vi "Calculate Indices.vi"(8 "Cursor.Cursor Y":dbl, 9 "Cursor.Cursor X":dbl, 10 "Vslow":dbl[](array[numeric]), 11 "Vfast":dbl[][](array[numeric])) -> (0 "Column":i32, 1 "Row":i32, 2 "Column Array":i32[](array[numeric]), 3 "Row Array":i32[](array[numeric]))   [LabVIEW 2016, in "Retrieve and Visualize.lvclass"]
uses:
  Retrieve and Visualize.lvclass
  <vilib>/gmath/NI_Gmath.lvlib
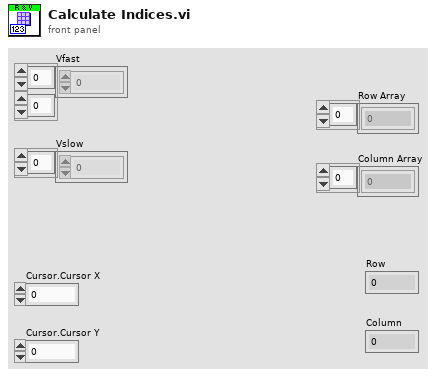
[diagram p1: front panel]
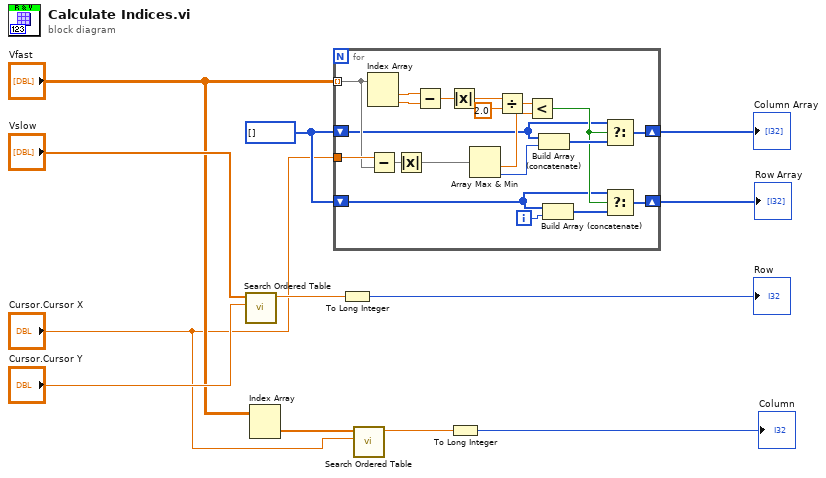
[diagram p0: block diagram]
diagram:
  w10 = i32[] []
  n1 = call <vilib>:"Search Ordered Table.vi"("x value"="Cursor.Cursor Y", "ordered x array"="Vslow") -> ("fractional index"=w6:dbl)  [unwired: 9 in]
  n2 = Index Array(array="Vfast") -> (element=w4:dbl[])  [unwired: 2 in]
  n3 = for {
    tunnel: "Vfast" -> [w15] mode=indexing
    tunnel: "Cursor.Cursor X" -> [w29]
    shift-right: [w21] -> w9
    shift-left: w10 -> [w14]
    shift-right: [w17] -> w8
    shift-left: w10 -> [w13]
    i -> [w20]
    n4 = Index Array(array=w15) -> (element #1=w28:dbl, element #2=w27:dbl)  [unwired: 2 in]
    n5 = Subtract(x=w29, y=w15) -> (x-y=w32:dbl[])
    n6 = Absolute Value(x=w32) -> (abs(x)=w31:dbl[])
    n7 = Subtract(x=w28, y=w27) -> (x-y=w30:dbl)
    n8 = Absolute Value(x=w30) -> (abs(x)=w26:dbl)
    n9 = Array Max & Min(array=w31) -> (min value=w23:dbl, min index (indices)=w16:i32)  [unwired: 2 out]
    n10 = Divide(x=w26, y=2.0) -> (x/y=w24:dbl)
    n11 = Less?(x=w24, y=w23) -> (x < y?=w18:bool)
    n12 = Build Array (concatenate)(w14, w16) -> (w22:i32[])
    n13 = Build Array (concatenate)(w13, w20) -> (w19:i32[])
    n14 = Select(t=w14, s=w18, f=w22) -> (s? t:f=w21:i32[])
    n15 = Select(t=w13, s=w18, f=w19) -> (s? t:f=w17:i32[])
  }
  "Column Array" <- w9
  "Row Array" <- w8
  n16 = To Long Integer(number=w6) -> (32bit integer=→"Row":i32)
  n17 = call <vilib>:"Search Ordered Table.vi"("x value"="Cursor.Cursor X", "ordered x array"=w4) -> ("fractional index"=w3:dbl)  [unwired: 9 in]
  n18 = To Long Integer(number=w3) -> (32bit integer=→"Column":i32)
